vi "Broadcast Self Test Result.vi"(8 "error in (no error)":errorcluster, 11 "Device Under Test in":refnum<class "Device Under Test.lvclass">) -> (0 "error out":errorcluster, 3 "Device Under Test out":refnum<class "Device Under Test.lvclass">)   [LabVIEW 2020, in "Device Under Test.lvclass"]
uses:
  Device Under Test.lvclass
  Device Under Test.lvclass/Device Under Test.ctl
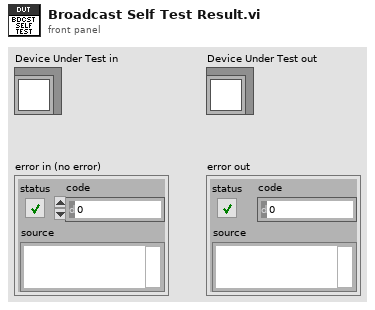
[diagram p1: front panel]
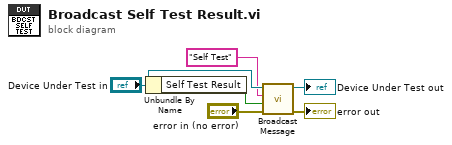
[diagram p0: block diagram]
diagram:
  n1 = Unbundle By Name("Device Under Test in") -> ("Self Test Result"=w4:bool)
  n2 = call-dynamic "Broadcast Message.vi"("error in (no error)"="error in (no error)", "Message Data"=w4, "Message"="Self Test", "Process In"="Device Under Test in") -> ("error out"=→"error out":errorcluster, "Process Out"=→"Device Under Test out":refnum<class "Device Under Test.lvclass">)  [unwired: 6 in]
